vi "LUT - Test Getter.vi"(8 "error in (no error)":errorcluster) -> (0 "error out":errorcluster)   [LabVIEW 2017]
uses:
  <vilib>/addons/_JKI Toolkits/Caraya/classes/Assert/Assert True.vi
  <vilib>/addons/_JKI Toolkits/Caraya/classes/Assert/Assert Equal Value and Type_Variant.vi
  <vilib>/addons/_JKI Toolkits/Caraya/classes/Assert/Assert False.vi
  <vilib>/addons/_JKI Toolkits/Caraya/classes/Test/Test.lvclass
  <vilib>/addons/_JKI Toolkits/Caraya/classes/Assert/Assert.lvclass
  src/LUT/LUT.lvclass
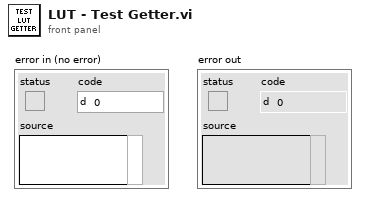
[diagram p1: front panel]
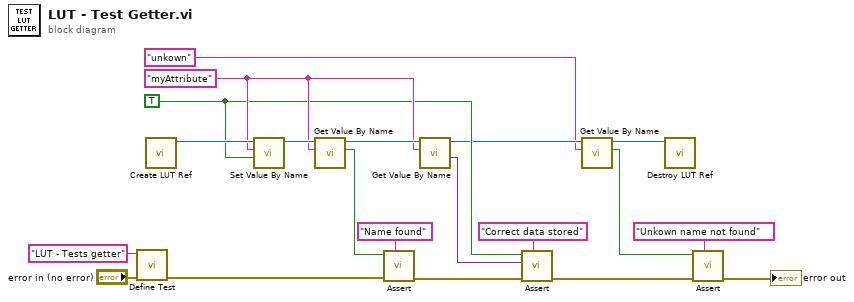
[diagram p0: block diagram]
diagram:
  w9 = TRUE
  w12 = "myAttribute"
  n1 = call <vilib>:"Define Test.vi"("error in (no error)"="error in (no error)", "Label (VI Title)"="LUT - Tests getter") -> ("error out"=w20:errorcluster)  [unwired: 9 in]
  n2 = call "Create LUT Ref.vi"() -> ("LUT out"=w17:refnum<class "LUT.lvclass">)  [unwired: 10 in, 1 out]
  n3 = call "Set Value By Name.vi"("Value"=w9, "Name"=w12, "LUT in"=w17) -> ("LUT out"=w16:refnum<class "LUT.lvclass">)  [unwired: 6 in, 2 out]
  n4 = call "Get Value By Name.vi"("Name"=w12, "LUT in"=w16) -> ("found?"=w14:bool, "LUT out"=w13:refnum<class "LUT.lvclass">)  [unwired: 6 in, 2 out]
  n5 = call-poly <vilib>:"Assert.vi"("Label"="Name found", "error in (no error)"=w20, "True?"=w14) -> ("error out"=w10:errorcluster)  [unwired: 8 in]
  n6 = call "Get Value By Name.vi"("Name"=w12, "LUT in"=w13) -> ("Value"=w8:variant, "LUT out"=w7:refnum<class "LUT.lvclass">)  [unwired: 6 in, 2 out]
  n7 = call-poly <vilib>:"Assert.vi"("Label"="Correct data stored", "error in (no error)"=w10, "Y"=w8, "X"=w9) -> ("error out"=w4:errorcluster)  [unwired: 7 in]
  n8 = call "Get Value By Name.vi"("Name"="unkown", "LUT in"=w7) -> ("found?"=w3:bool, "LUT out"=w1:refnum<class "LUT.lvclass">)  [unwired: 6 in, 2 out]
  n9 = call "Destroy LUT Ref.vi"("LUT in"=w1) -> ()  [unwired: 10 in, 1 out]
  n10 = call-poly <vilib>:"Assert.vi"("Label"="Unkown name not found", "error in (no error)"=w4, "False?"=w3) -> ("error out"=→"error out":errorcluster)  [unwired: 8 in]
